vi "TestConnection.vi"(7 "LabVIEW Web Service Request":refnum<class "Web Request.lvclass">) -> ()   [LabVIEW 2017]
uses:
  <vilib>/wsapi/Web Request.lvclass
  <vilib>/addons/InsightCM/MessageBus/Base/controls/ConnectionInfo.ctl
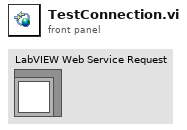
[diagram p1: front panel]
types:
  T1 = typedef "ConnectionInfo.ctl" = cluster{"ClientName":string, "TransceiverHost":string, "TransceiverPort":u16, "Password":string}
  T2 = typedef "TcpMessageReference.ctl" = refnum<data-value>
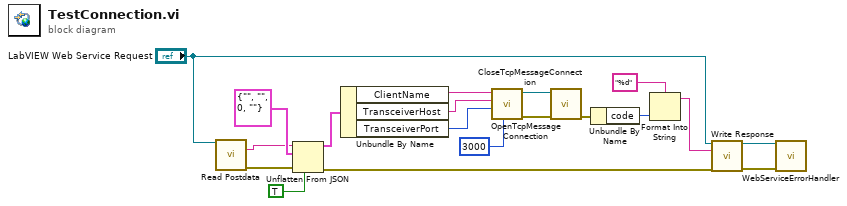
[diagram p0: block diagram]
diagram:
  n1 = call <vilib>:"Read Postdata.vi"("LabVIEW Web Service Request"="LabVIEW Web Service Request") -> ("postdata"=w15:string, "error out"=w14:errorcluster)  [unwired: 12 in, 1 out]
  n2 = Unflatten From JSON(JSON string=w15, type and defaults=T1 {"ClientName"="", "TransceiverHost"="", "TransceiverPort"=0, "Password"=""} ("ConnInfo"), default null elements? (F)=TRUE, error in (no error)=w14) -> (value=w11:T1, error out=w13:errorcluster)  [unwired: 3 in]
  n3 = Unbundle By Name(w11) -> ("ClientName"=w10:string, "TransceiverHost"=w9:string, "TransceiverPort"=w8:u16)
  n4 = call <vilib>:"OpenTcpMessageConnection.vi"("timeout (ms)"=3000, "Port"=w8, "Hostname"=w9, "ClientName"=w10) -> ("error out"=w5:errorcluster, "connection ID out"=w6:T2)  [unwired: 6 in]
  n5 = call <vilib>:"CloseTcpMessageConnection.vi"("error in (no error)"=w5, "connection ID in"=w6) -> ("error out"=w4:errorcluster)  [unwired: 9 in]
  n6 = Unbundle By Name(w4) -> ("code"=w3:i32)
  n7 = Format Into String(format string="%d", w3) -> (resulting string=w2:string)  [unwired: 2 in, 1 out]
  n8 = call <vilib>:"Write Response.vi"("LabVIEW Web Service Request"="LabVIEW Web Service Request", "response string"=w2, "error in (no error)"=w13) -> ("LabVIEW Web Service Request out"=w18:refnum<class "Web Request.lvclass">, "error out"=w19:errorcluster)  [unwired: 11 in]
  n9 = call "WebServiceErrorHandler.vi"("LabVIEW Web Service Request"=w18, "error in (no error)"=w19) -> ()  [unwired: 12 in, 2 out]
